vi "Set_DAQmxTask + Name.vi"(8 "error in (no error)":errorcluster, 9 "Task name":string, 10 "DAQmxTask.lvclass":refnum<class "DAQmxTask.lvclass">, 11 "DAQmxTaksContainer_General in":refnum<class "DAQmxTaksContainer_General.lvclass">) -> (0 "error out":errorcluster, 3 "DAQmxTaksContainer_General out":refnum<class "DAQmxTaksContainer_General.lvclass">)   [LabVIEW 2015, in "DAQmxTaksContainer_General.lvclass"]
uses:
  DAQmxTaksContainer_General.lvclass
  DAQmxTask.lvclass
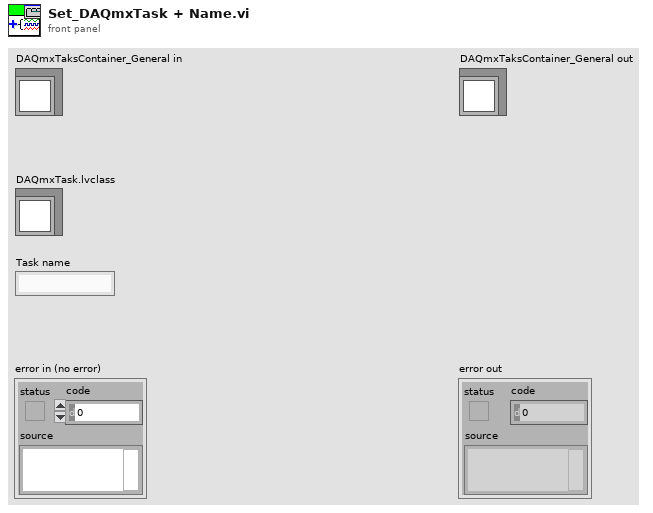
[diagram p1: front panel]
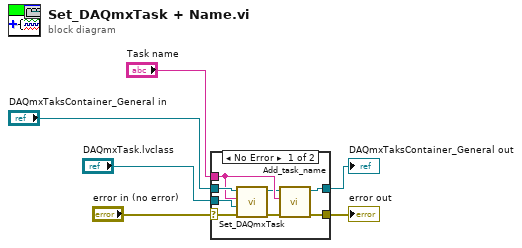
[diagram p0: block diagram]
diagram:
  n1 = case shown="No Error" "error in (no error)" {
    selector: "error in (no error)" -> [w11 w16]
    tunnel: [w13 w16] -> w5
    tunnel: [w14 w15] -> w3
    tunnel: "DAQmxTaksContainer_General in" -> [w12 w15]
    tunnel: "DAQmxTask.lvclass" -> [w10 _]
    tunnel: "Task name" -> [w9 _]
    frame No Error {
      n2 = call "Set_DAQmxTask.vi"("error in (no error)"=w11, "DAQmxTask"=w10, "Task name"=w9, "DAQmxTaksContainer_General in"=w12) -> ("error out"=w7:errorcluster, "DAQmxTaksContainer_General out"=w8:refnum<class "DAQmxTaksContainer_General.lvclass">)  [unwired: 6 in]
      n3 = call "Add_task_name.vi"("error in (no error)"=w7, "new name of task"=w9, "DAQmxTaksContainer_General in"=w8) -> ("error out"=w13:errorcluster, "DAQmxTaksContainer_General out"=w14:refnum<class "DAQmxTaksContainer_General.lvclass">)  [unwired: 7 in]
    }
    frame Error {
    }
  }
  "error out" <- w5
  "DAQmxTaksContainer_General out" <- w3
